vi "Path String.vi"(11 "URI in":refnum<class "URI.lvclass">) -> (2 "Path String":string, 3 "URI out":refnum<class "URI.lvclass">)   [LabVIEW 2020, in "URI.lvlib" / "URI.lvclass"]
uses:
  URI.lvclass
  URI.lvclass/URI.ctl
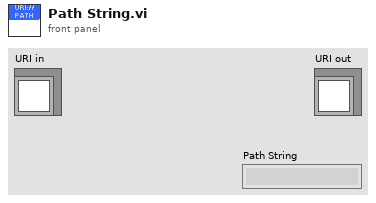
[diagram p1: front panel]
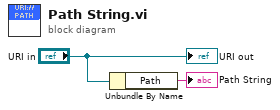
[diagram p0: block diagram]
diagram:
  n1 = Unbundle By Name("URI in") -> ("Path"=→"Path String":string)
  "URI out" <- "URI in"
